vi "qTWS.vi"(0 "System no.":i32=1 min=1 max=4 step=1, 2 "TriggerOut to query":i32[](array[numeric]), 3 "Without parameter?":bool, 5 "error in":errorcluster, 6 "Xo":i32, 7 "N":i32=100, 8 "Nmax":i32=1024) -> (14 "Data":dbl[][](array[numeric]) format="%.2f", 15 "TWS? string":string, 19 "error out":errorcluster)   [LabVIEW 2026]
doc: "Returns trigger points set by TWS. N must be less than or equal to Nmax. For large N values, communication timeout must be set long enough, otherwise a comm. error may occur.\n\nE-517, E-518: Nmax = 8192.\nE-712: Nmax = 262,144.\nE-725, E-727: Nmax = 262,144.\nE-753: Nmax = 262,144. \nE-754: Nmax = 1,048,576."
panel:
  # "Returns trigger points set by TWS. N must be less than or equal to Nmax. For large N values, \ncommunication timeout must be set long enough, otherwise a comm.error may occur."
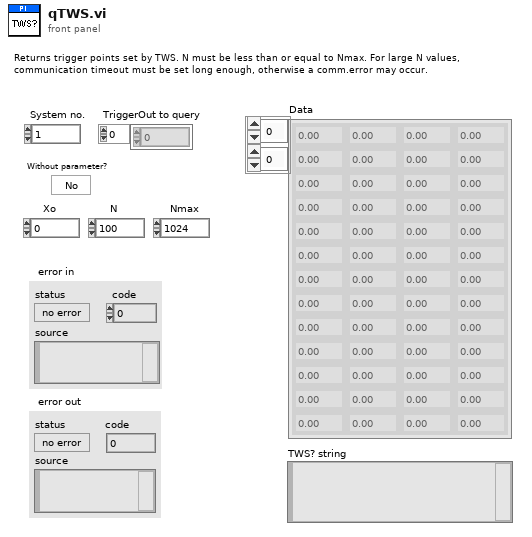
[diagram p1: front panel]
types:
  T1 = cluster{"Read (F)/Write":bool, "Path":path, "Datastream":string, "ArrayName":string}
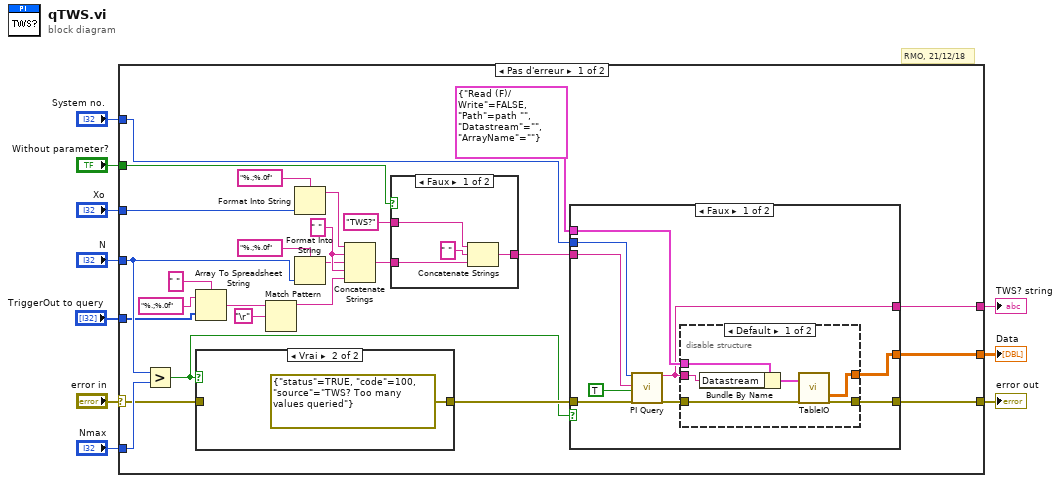
[diagram p0: block diagram]
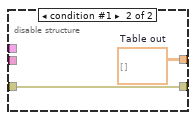
[diagram p3: hidden frame]
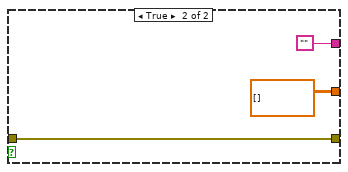
[diagram p4: hidden frame]
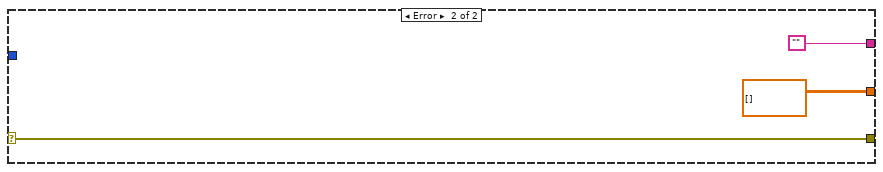
[diagram p6: hidden frame]
diagram:
  # "RMO, 21/12/18"
  n1 = case shown="Pas d'erreur" "error in" {
    selector: "error in" -> [w11 w64]
    tunnel: "System no." -> [w34 _]
    tunnel: "TriggerOut to query" -> [w17 _]
    tunnel: [w30 w64] -> w9
    tunnel: [w29 dbl[][] [] ("Table out")] -> w5
    tunnel: "N" -> [w24 _]
    tunnel: "Xo" -> [w27 _]
    tunnel: "Nmax" -> [w25 _]
    tunnel: "Without parameter?" -> [w13 _]
    tunnel: [w12 ""] -> w2
    frame No Error {
      w26 = " "
      n2 = Greater?(x=w24, y=w25) -> (0:w31:bool)
      n3 = Array To Spreadsheet String(delimiter (Tab)=" ", array=w17, 3:"%.;%.0f" ("Format String")) -> (spreadsheet string=w16:string)
      n4 = case shown="Vrai" w31 {
        tunnel: [w62 errorcluster {"status"=TRUE, "code"=100, "source"="TWS? Too many values queried"} ("error out")] -> w32
        tunnel: w11 -> [w62 _]
        frame False {
        }
        frame True {
        }
      }
      n5 = Match Pattern(string=w16, regular expression="\r") -> (before substring=w15:string)  [unwired: 4 out]
      n6 = Format Into String(format string="%.;%.0f" ("Format String"), w27) -> (resulting string=w22:string)  [unwired: 2 in, 1 out]
      n7 = Format Into String(format string="%.;%.0f" ("Format String"), w24) -> (resulting string=w21:string)  [unwired: 2 in, 1 out]
      n8 = Concatenate Strings(w22, w26, w21, w26, w15) -> (w14:string)
      n9 = case shown="Faux" w13 {
        tunnel: "TWS?" -> [w40 w41]
        tunnel: [w39 w41] -> w35
        tunnel: w14 -> [w38 _]
        frame False {
          n10 = Concatenate Strings(w40, " " ("Substring"), w38) -> (w39:string)
        }
        frame True {
        }
      }
      n11 = case shown="Faux" w31 {
        tunnel: w35 -> [w49 _]
        tunnel: w34 -> [w48 _]
        tunnel: w32 -> [w45 w61]
        tunnel: [w44 w61] -> w30
        tunnel: [w46 dbl[][] [] ("Table out")] -> w29
        tunnel: T1 {"Read (F)/Write"=FALSE, "Path"=path "", "Datastream"="", "ArrayName"=""} ("IOSource") -> [w47 _]
        tunnel: [w42 ""] -> w12
        frame False {
          n12 = call "PI Query.vi"("System no."=w48, "String to send"=w49, "Attach termination char.?"=TRUE ("Attach Linefeed?"), "error in"=w45) -> ("String read"=w42:string, "error out"=w43:errorcluster)  [unwired: 3 in, 11 out]
          n13 = disable-structure shown="Default" {
            disable-tunnel: w42 -> [w56 _]
            disable-tunnel: w47 -> [w55 _]
            disable-tunnel: [w53 w58] -> w46
            disable-tunnel: w43 -> [w52 w57]
            disable-tunnel: [w51 w57] -> w44
            frame condition #0 (active) {
              n14 = Bundle By Name(cluster=w55, "Datastream"=w56) -> (w54:T1)
              n15 = call "TableIO.vi"("IOSource"=w54, "error in"=w52) -> ("Table out"=w53:dbl[][], "error out"=w51:errorcluster)  [unwired: 4 in, 12 out]
            }
            frame condition #1 {
              w58 = dbl[][] []  # Table out
            }
          }
        }
        frame True {
        }
      }
    }
    frame Error {
    }
  }
  "error out" <- w9
  "Data" <- w5
  "TWS? string" <- w2
